vi "writeSDOU16.vi"(6 "object sub-index (0)":u8 format="%x", 7 "object index":u16 format="%x", 8 "error in (no error)":errorcluster, 9 "interface object in":refnum<k20>, 10 "inputNumber":u16, 11 "MotorControllerClass in":refnum<class "MotorControllerClass.lvclass">) -> (0 "error out":errorcluster, 1 "completion code":u32, 2 "interface object out":refnum<k20>, 3 "MotorControllerClass out":refnum<class "MotorControllerClass.lvclass">)   [LabVIEW 2018, in "MotorControllerClass.lvclass"]
uses:
  BMS/MotorControllerClass.lvclass
  <vilib>/CANopenLib/CANOPEN.llb/CANopen SDO Create.vi
  <vilib>/CANopenLib/CANOPEN.llb/CANopen SDO Write [U16].vi
  <vilib>/CANopenLib/CANOPEN.llb/CANopen SDO Close.vi
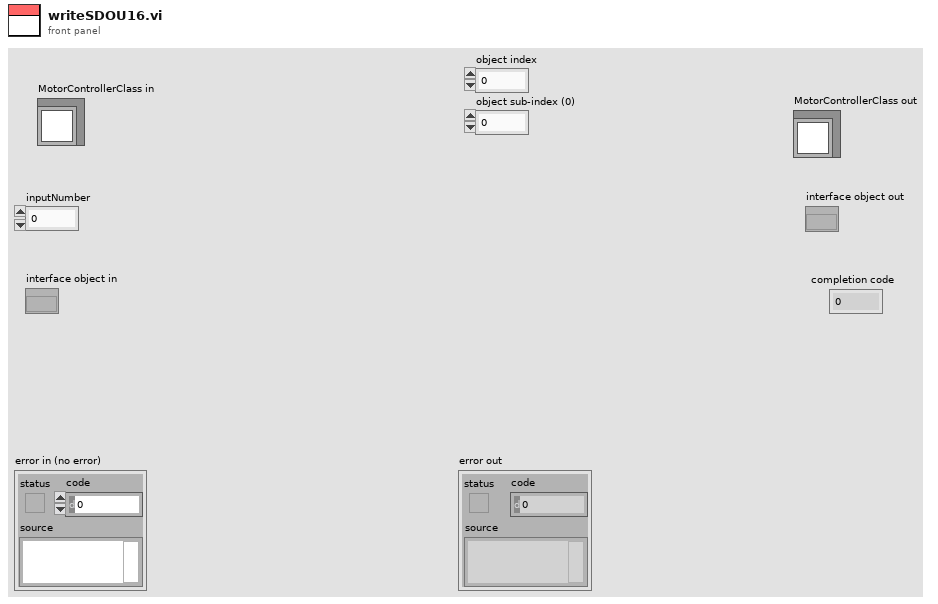
[diagram p1: front panel]
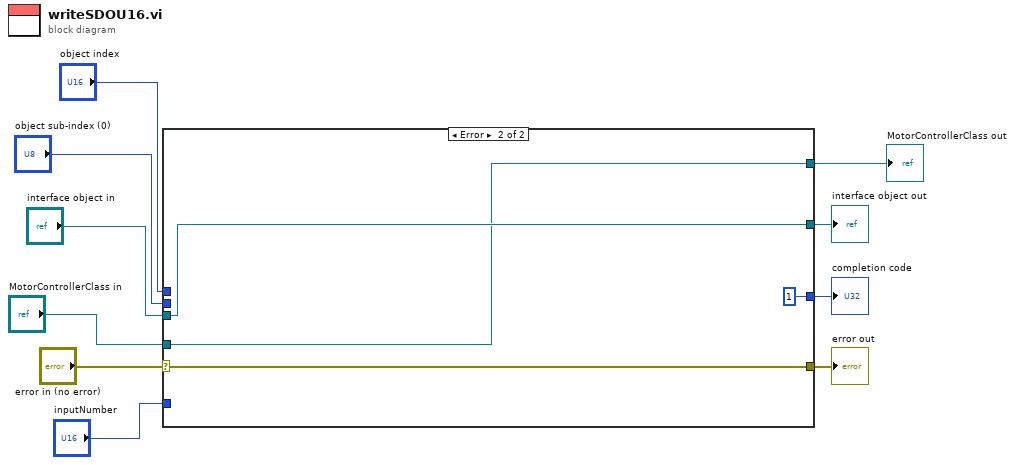
[diagram p0: block diagram]
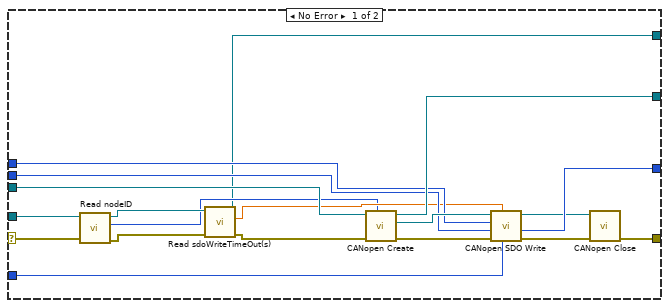
[diagram p2: hidden frame]
diagram:
  n1 = case shown="Error" "error in (no error)" {
    selector: "error in (no error)" -> [w18 w33]
    tunnel: [w21 w33] -> w9
    tunnel: [w29 w31] -> w8
    tunnel: "interface object in" -> [w28 w31]
    tunnel: "object index" -> [w26 _]
    tunnel: "object sub-index (0)" -> [w25 _]
    tunnel: "inputNumber" -> [w24 _]
    tunnel: [w23 u32 1 ("completion code")] -> w3
    tunnel: "MotorControllerClass in" -> [w14 w30]
    tunnel: [w11 w30] -> w1
    frame No Error {
      n2 = call-dynamic "Read nodeID.vi"("error in (no error)"=w18, "MotorControllerClass in"=w14) -> ("error out"=w17:errorcluster, "nodeID"=w12:u8, "MotorControllerClass out"=w13:refnum<class "MotorControllerClass.lvclass">)  [unwired: 7 in]
      n3 = call-dynamic "Read sdoWriteTimeOut(s).vi"("error in (no error)"=w17, "MotorControllerClass in"=w13) -> ("error out"=w16:errorcluster, "sdoWriteTimeOut(s)"=w15:dbl, "MotorControllerClass out"=w11:refnum<class "MotorControllerClass.lvclass">)  [unwired: 7 in]
      n4 = call-poly <vilib>:"CANopen Create.vi"("node-ID"=w12, "error in (no error)"=w16, "interface object in"=w28) -> ("error out"=w19:errorcluster, "SDO object out"=w27:refnum<k20>, "interface object out"=w29:refnum<k20>)  [unwired: 6 in]
      n5 = call-poly <vilib>:"CANopen SDO Write.vi"("U16 data"=w24, "timeout (1s)"=w15, "error in (no error)"=w19, "object sub-index (0)"=w25, "object index"=w26, "SDO object in"=w27) -> ("error out"=w22:errorcluster, "completion code"=w23:u32, "SDO object out"=w20:refnum<k20>)  [unwired: 3 in]
      n6 = call-poly <vilib>:"CANopen Close.vi"("error in (no error)"=w22, "SDO object in"=w20) -> ("error out"=w21:errorcluster)  [unwired: 9 in]
    }
    frame Error {
    }
  }
  "error out" <- w9
  "interface object out" <- w8
  "completion code" <- w3
  "MotorControllerClass out" <- w1
